vi "Keithley 2600 IV sweep.vi"(0 "VISA resource name":refnum<visa-resource-name>, 1 "Filter Count (1)":i32=1, 2 "Settling (ms)":u32=500, 3 "Current limit (0.1)":dbl=0.1, 5 "Node In":string, 7 "Channel (Channel A)":T1, 9 "Voltage points":dbl[](array[numeric]), 11 "error in (no error)":errorcluster, 12 "Stop occurrence":refnum<k4>, 13 "XY Graph to update":refnum<vi>, 14 "Status String Reference":refnum<vi>) -> (4 "VISA resource name out":refnum<visa-resource-name>, 6 "Current points":dbl[](array[numeric]), 8 "Voltage points (Collected)":dbl[](array[numeric]), 15 "error out":errorcluster)   [LabVIEW 2019]
uses:
  <instrlib>/Keithley 2600 Series/Public/Channel.ctl
  <instrlib>/Keithley 2600 Series/Keithley 2600 Series.lvlib
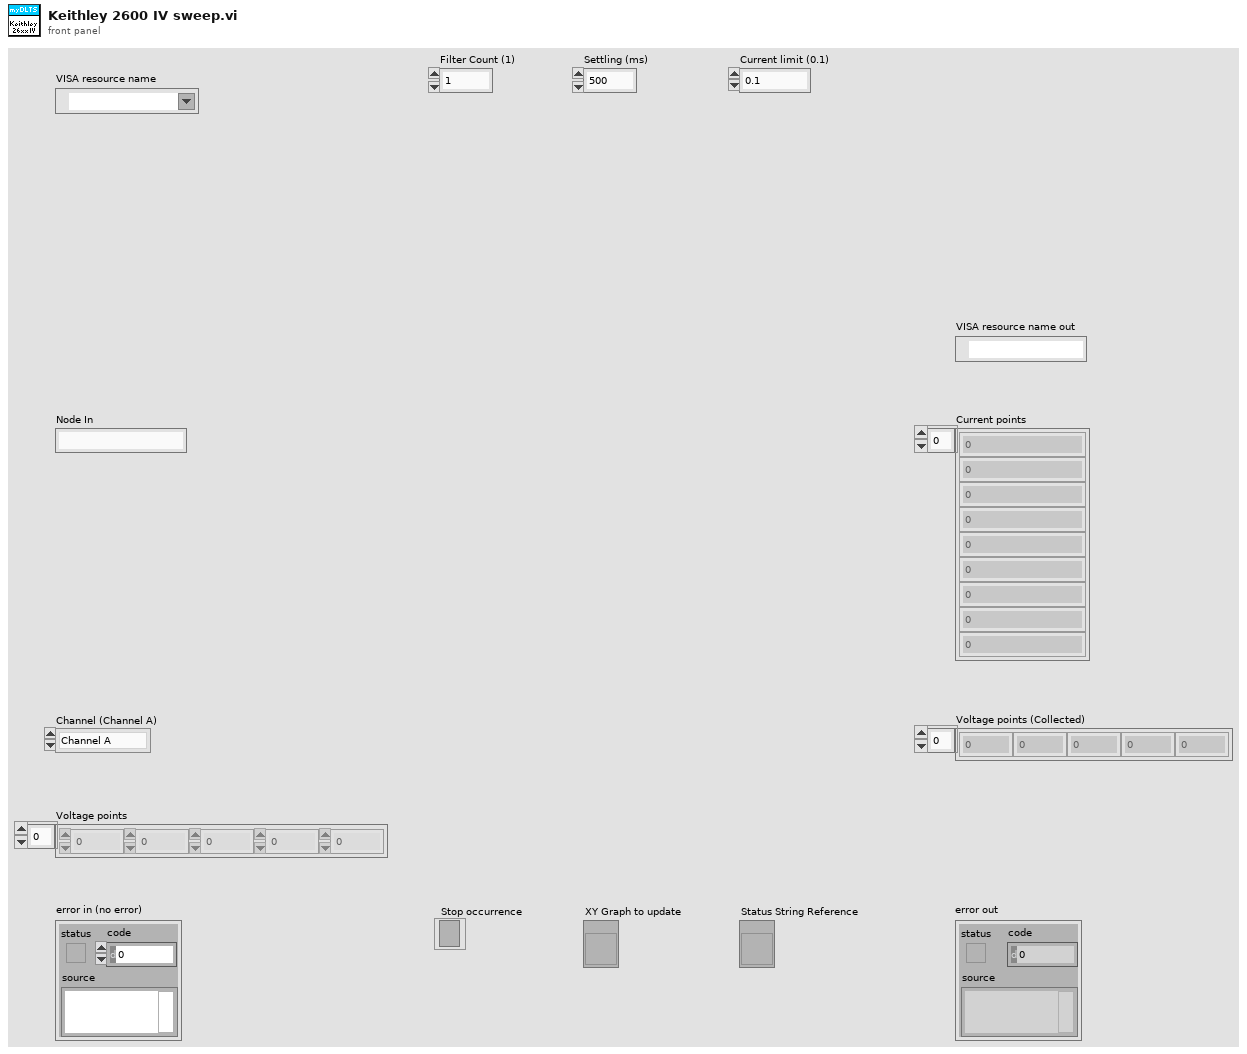
[diagram p1: front panel]
types:
  T1 = typedef "Keithley 2600 Series.lvlib/Channel.ctl" = enum32{"Channel A", "Channel B"}
  T2 = enum32{"Current", "Voltage", "Resistance", "Power"}
  T3 = enum32{"Current", "Voltage", "IV", "Resistance", "Power"}
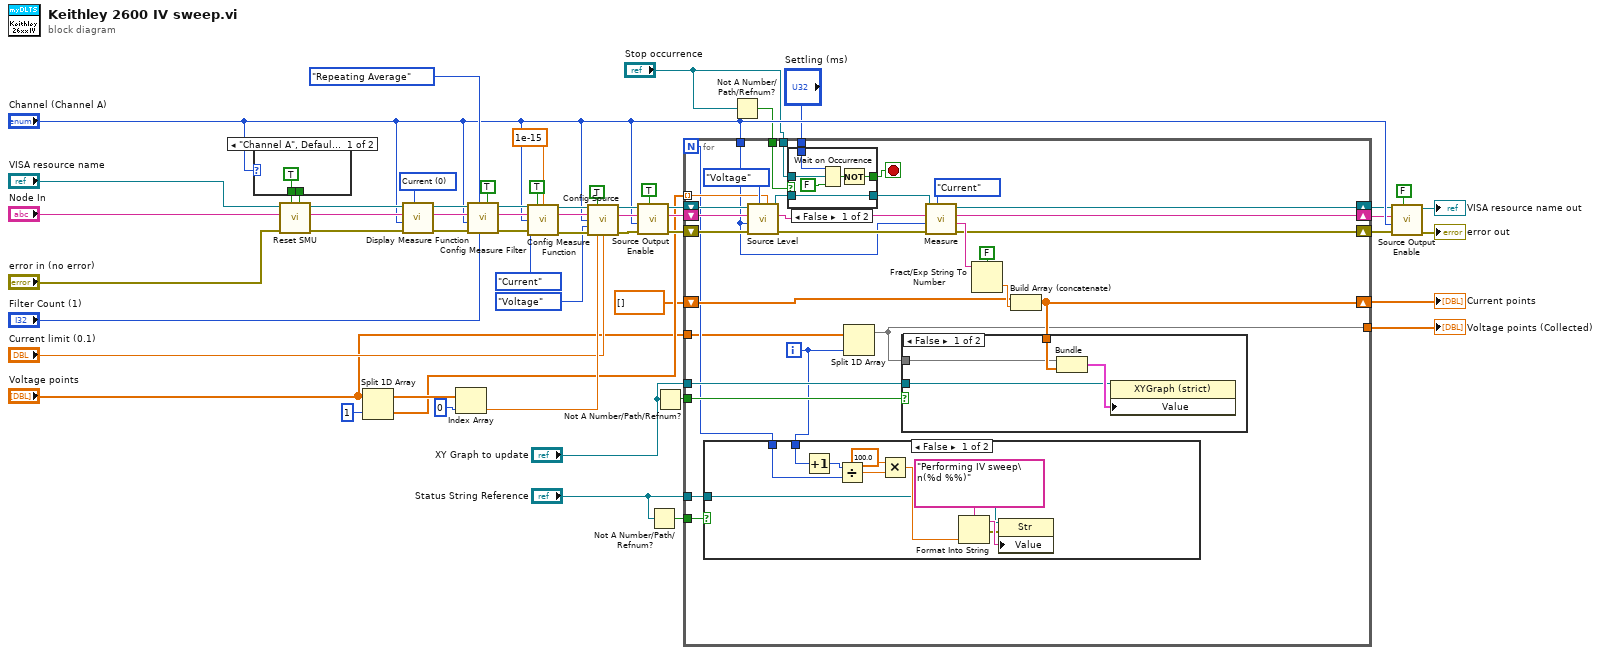
[diagram p0: block diagram]
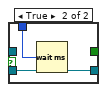
[diagram p2: hidden frame]
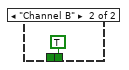
[diagram p5: hidden frame]
diagram:
  w33 = u16 0 items=["Current", "Voltage", "Resistance", "Power"] ("Function (Current)")
  n1 = case shown="\"Channel A\", Default" "Channel (Channel A)" {
    tunnel: [TRUE ("SMU A (No)") _] -> w57
    tunnel: [_ TRUE ("SMU A (No)")] -> w56
    frame "Channel A", Default {
    }
    frame "Channel B" {
    }
  }
  n2 = call <instrlib>:"Reset SMU.vi"("SMU B (No)"=w56, "SMU A (No)"=w57, "error in (no error)"="error in (no error)", "Node In"="Node In", "VISA resource name"="VISA resource name") -> ("error out"=w37:errorcluster, "Node Out"=w38:string, "VISA resource name out"=w39:refnum<visa-resource-name>)  [unwired: 3 in, 1 out]
  n3 = Split 1D Array(array="Voltage points", index=1) -> (first subarray=w31:dbl[], second subarray=w13:dbl[])
  n4 = call <instrlib>:"Display Measure Function.vi"("Function (Current)"=w33, "error in (no error)"=w37, "Channel (Channel A)"="Channel (Channel A)", "Node In"=w38, "VISA resource name"=w39) -> ("error out"=w36:errorcluster, "Node Out"=w35:string, "VISA resource name out"=w34:refnum<visa-resource-name>)  [unwired: 3 in, 1 out]
  n5 = Index Array(array=w31, index=0) -> (element=w30:dbl)
  n6 = call <instrlib>:"Config Measure Filter.vi"("On/Off (Off)"=TRUE, "Count (1)"="Filter Count (1)", "Filter Type (Moving Average)"=enum32{"Moving Average", "Repeating Average"}."Repeating Average", "error in"=w36, "Channel (Channel A)"="Channel (Channel A)", "Node In"=w35, "VISA resource name"=w34) -> ("error out"=w53:errorcluster, "Node Out"=w52:string, "VISA resource name out"=w54:refnum<visa-resource-name>)  [unwired: 1 in, 1 out]
  n7 = call <instrlib>:"Config Measure Function.vi"("VISA resource name"=w54, "Autorange (On)"=TRUE, "Low Range (1.000)"=1e-15, "Node In"=w52, "Channel (Channel A)"="Channel (Channel A)", "Function (Current)"=T2."Current", "error in"=w53) -> ("VISA resource name out"=w48:refnum<visa-resource-name>, "Node Out"=w44:string, "error out"=w47:errorcluster)  [unwired: 5 in, 1 out]
  n8 = call <instrlib>:"Config Source.vi"("VISA resource name"=w48, "Autorange (On)"=TRUE, "Node In"=w44, "Channel (Channel A)"="Channel (Channel A)", "Function (Current)"=enum32{"Current", "Voltage"}."Voltage", "error in"=w47, "Level (0.000)"=w30, "Limit (0.1)"="Current limit (0.1)") -> ("VISA resource name out"=w43:refnum<visa-resource-name>, "Node Out"=w41:string, "error out"=w42:errorcluster)  [unwired: 4 in, 1 out]
  n9 = call <instrlib>:"Source Output Enable.vi"("Output (Off)"=TRUE, "error in (no error)"=w42, "Channel (Channel A)"="Channel (Channel A)", "Node In"=w41, "VISA resource name"=w43) -> ("error out"=w27:errorcluster, "Node Out"=w28:string, "VISA resource name out"=w24:refnum<visa-resource-name>)  [unwired: 3 in, 1 out]
  n10 = Not A Number/Path/Refnum?(number/path/refnum="Status String Reference") -> (NaN/Path/Refnum?=w11:bool)
  n11 = Not A Number/Path/Refnum?(number/path/refnum="XY Graph to update") -> (NaN/Path/Refnum?=w12:bool)
  n12 = Not A Number/Path/Refnum?(number/path/refnum="Stop occurrence") -> (NaN/Path/Refnum?=w9:bool)
  n13 = for {
    N -> [w69]
    tunnel: "Channel (Channel A)" -> [w81]
    tunnel: w13 -> [w84] mode=indexing
    shift-right: [w77] -> w22
    shift-left: w27 -> [w89]
    shift-right: [w78] -> w20
    shift-left: w24 -> [w88]
    shift-right: [w79] -> w21
    shift-left: w28 -> [w87]
    tunnel: "Settling (ms)" -> [w65]
    shift-right: [w74] -> w19
    shift-left: dbl[] [] -> [w75]
    tunnel: "Voltage points" -> [w61]
    tunnel: "XY Graph to update" -> [w73]
    tunnel: w12 -> [w72]
    tunnel: w11 -> [w71]
    tunnel: "Status String Reference" -> [w70]
    tunnel: w9 -> [w63]
    tunnel: "Stop occurrence" -> [w62]
    tunnel: [w60] -> w3
    i -> [w68]
    stop <- w64 stop-if-true
    n14 = case shown="False" w71 {
      tunnel: w70 -> [w99 _]
      tunnel: w69 -> [w106 _]
      tunnel: w68 -> [w108 _]
      frame False {
        n15 = Increment(x=w108) -> (x+1=w107:i32)
        n16 = Divide(x=w107, y=w106) -> (x/y=w105:dbl)
        n17 = Multiply(x=100.0, y=w105) -> (x*y=w100:dbl)
        n18 = Format Into String(format string="Performing IV sweep\n(%d %%)", w100) -> (resulting string=w103:string, error out=w102:errorcluster)  [unwired: 2 in]
        n19 = property class="Str"(reference=w99, error in=w102, "Value"=w103) -> ()  [unwired: 2 out]
      }
      frame True {
      }
    }
    n20 = call <instrlib>:"Source Level.vi"("Level (0.000)"=w84, "Function (Current)"=enum32{"Current", "Voltage"}."Voltage", "error in (no error)"=w89, "Channel (Channel A)"=w81, "Node In"=w87, "VISA resource name"=w88) -> ("error out"=w82:errorcluster, "Node Out"=w83:string, "VISA resource name out"=w67:refnum<visa-resource-name>)  [unwired: 2 in, 1 out]
    n21 = case shown="False" w63 {
      tunnel: [w95 _] -> w64
      tunnel: w65 -> [w94 w98]
      tunnel: w62 -> [w93 _]
      tunnel: w67 -> [w92 w97]
      tunnel: [w92 w97] -> w66
      frame False {
        n22 = Wait on Occurrence(1:FALSE ("ignore previous (T)"), 2:w93, 3:w94) -> (0:w96:bool)
        n23 = Not(x=w96) -> (.not. x?=w95:bool)
      }
      frame True {
        n24 = Wait (ms)(milliseconds to wait=w98) -> ()  [unwired: 1 out]
      }
    }
    n25 = Split 1D Array(array=w61, index=w68) -> (first subarray=w60:dbl[])  [unwired: 1 out]
    n26 = call <instrlib>:"Measure.vi"("Function (Current)"=T3."Current", "error in (no error)"=w82, "Channel (Channel A)"=w81, "Node In"=w83, "VISA resource name"=w66) -> ("error out"=w77:errorcluster, "Output"=w80:string, "Node Out"=w79:string, "VISA resource name out"=w78:refnum<visa-resource-name>)  [unwired: 2 in, 1 out]
    n27 = Fract/Exp String To Number(use system decimal point (T)=FALSE, string=w80) -> (number=w76:dbl)  [unwired: 2 in, 1 out]
    n28 = Build Array (concatenate)(w75, w76) -> (w74:dbl[])
    n29 = case shown="False" w72 {
      tunnel: w74 -> [w112 _]
      tunnel: w73 -> [w110 _]
      tunnel: w60 -> [w109 _]
      frame False {
        n30 = Bundle(w109, w112) -> (w111:cluster{dbl[], dbl[]})  [unwired: 1 in]
        n31 = property on="Property Node" class="XYGraph (strict)"(reference=w110, "Value"=w111) -> ()  [unwired: 1 in, 2 out]
      }
      frame True {
      }
    }
  }
  "Current points" <- w19
  "Voltage points (Collected)" <- w3
  n32 = call <instrlib>:"Source Output Enable.vi"("Output (Off)"=FALSE, "error in (no error)"=w22, "Channel (Channel A)"="Channel (Channel A)", "Node In"=w21, "VISA resource name"=w20) -> ("error out"=→"error out":errorcluster, "VISA resource name out"=→"VISA resource name out":refnum<visa-resource-name>)  [unwired: 3 in, 2 out]
